vi "Engineering mode.vi"() -> ()   [LabVIEW 2017]
uses:
  Ctrls/TesterInfo.ctl
  Ctrls/HD Config.ctl
  Ctrls/AllControls.ctl
  Ctrls/Position Config.ctl
  <vilib>/Utility/miscctls.llb/LVRowAndColumnTypeDef.ctl
  DIPC 692 Daemon API/typdef/destination.ctl
  DIPC 692 Daemon API/typdef/device_mode.ctl
  ComVIS/Files/Ini/WriteIniFiles_ByVarient.vi
  <vilib>/Utility/file.llb/Write Delimited Spreadsheet (string).vi
  HardWare/ADLINK/IO/Adlink IO/Adlink IO.lvlib
panel:
  in  "Data":string
  out "Size":i32
  in  "AllControls":T1
  in  "Production Mode":bool
  out "Save_status":string
  in  "Selecttion":T2(tab)
  in  "HD Config Save":bool
  in  "HD Config":T3
  in  "SW Config Save":bool
  in  "TesterInfo":T4
  in  "Table":T5(tab)
  in  "Table_Data":string[][](table)
  in  "Title_Data":string[][](table)
  in  "Config":string[][](table)
  in  "SKU_Table":string[][](table)
  in  "Debug":T6(tab)
  in  "IO":i32(listbox)
  in  "Reset":bool
  in  "Set_MaxSpeed":u32
  in  "Set_Speed":bool
  in  "Set_MoveSpeed":u16 max=100
  in  "Stop":bool
  in  "Servo_Off":bool
  in  "Servo_On":bool
  in  "Position Config":T7
  in  "PositionSelect":T8(ring)
  in  "Home":bool
  in  "Position Config Save":bool
  in  "GoPosition":bool
  in  "Zero pressure":bool
  out "Status":string
  out "Units":string
  out "Pressure":string
  in  "FCO Model5_Read":bool
  out "FCO Data":string
  in  "Relay_ON/OFF":bool
  in  "DC_Power_ON/OFF":bool
  in  "DC_Set":bool
  in  "DC":bool
  out "DC Power Data":string
  in  "Voltage":dbl min=0.0 max=25.0
  in  "Current":dbl min=0.0 max=48.0
  out "Measurement":dbl[](array[numeric])
  in  "PW3336":bool
  out "PW3336 Data":string
  out "Atmospheric Pressure":dbl
  in  "Lefoo":bool
  out "Lefoo Data":string
  out "UID":string
  out "temperature":dbl
  out "humidity":dbl
  in  "Read_NFC":bool
  out "DataTag":string
  out "Data Return":string
  in  "Set EOL":bool
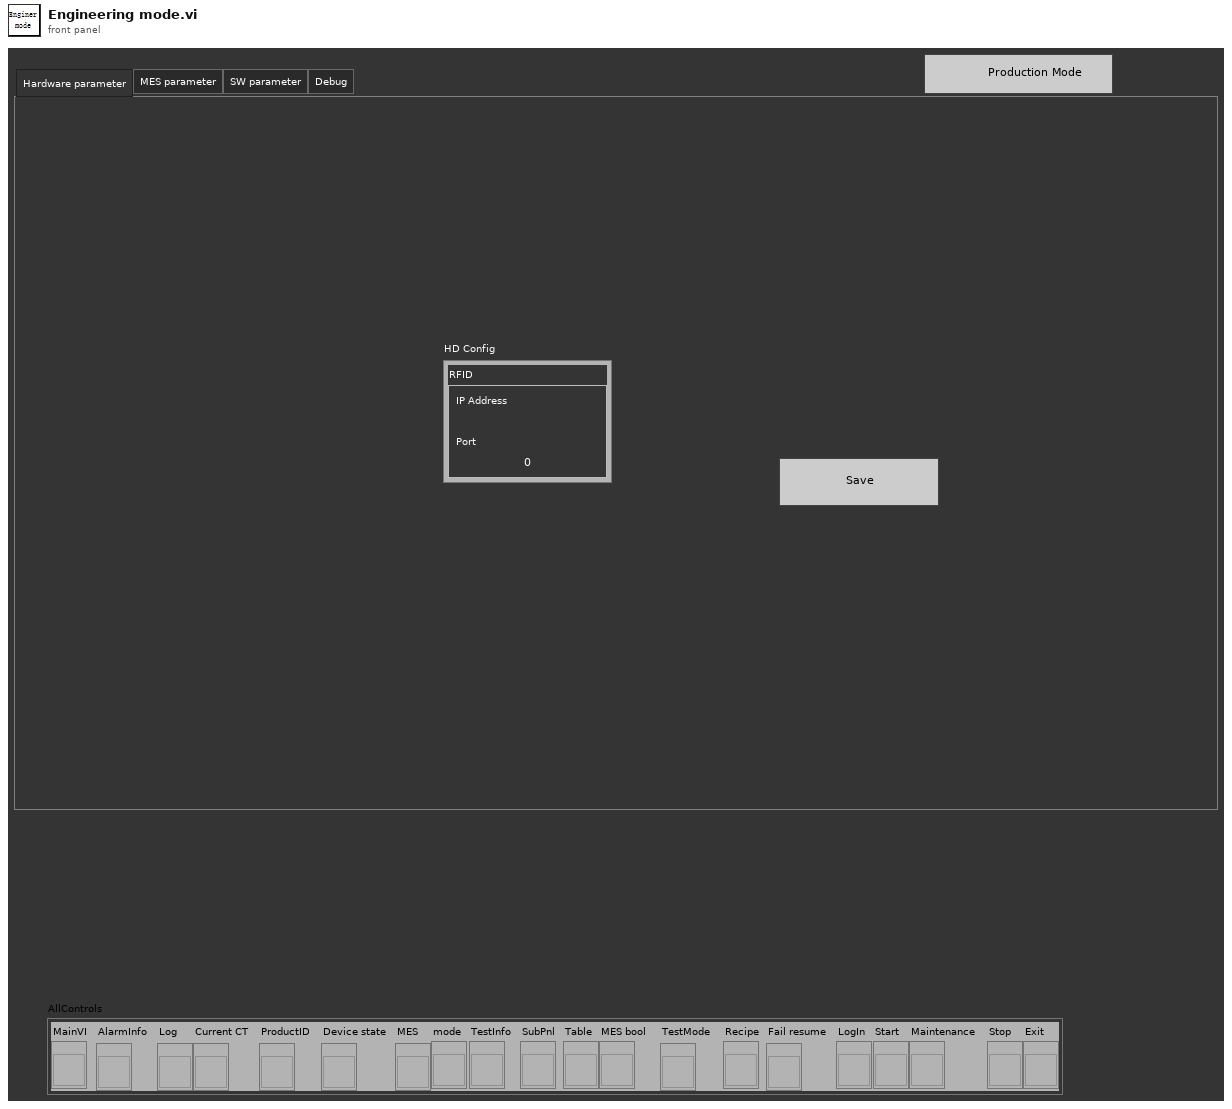
[diagram p1: front panel]
types:
  T1 = typedef "AllControls.ctl" = cluster{"MainVI":refnum<vi>, "AlarmInfo":refnum<vi>, "Log":refnum<vi>, "Current CT":refnum<vi>, "ProductID":refnum<vi>, "Device state":refnum<vi>, "MES":refnum<vi>, "mode":refnum<vi>, "TestInfo":refnum<vi>, "SubPnl":refnum<vi>, "Table":refnum<vi>, "MES bool":refnum<vi>, "TestMode":refnum<vi>, "Recipe":refnum<vi>, "Fail resume":refnum<vi>, "LogIn":refnum<vi>, "Start":refnum<vi>, "Maintenance":refnum<vi>, "Stop":refnum<vi>, "Exit":refnum<vi>}
  T2 = enum32{"Hardware parameter", "MES parameter", "SW parameter", "Debug"}
  T3 = typedef "HD Config.ctl" = cluster{" PC":cluster{"PC Address":u8[], "PC Port":i32}, "FCO":cluster{"COM":refnum<visa-resource-name>, "Baudrate":u32}, "DC Power ":cluster{"COM":refnum<visa-resource-name>, "Baudrate":u32}, "PW3336":cluster{"COM":refnum<visa-resource-name>, "Baudrate":u32}, "Lefoo":cluster{"COM":refnum<visa-resource-name>, "Baudrate":u32}, "AI Model":cluster{"COM":refnum<visa-resource-name>, "Baudrate":u32}, "DIPC":cluster{"COM":refnum<visa-resource-name>}, "RFID":cluster{"IP Address":string, "Port":u16, "Retry":u16}, "Motor":cluster{"COM":refnum<visa-resource-name>, "Baudrate":u32}, "Fail_resume_mode":bool, "GRR":bool}
  T4 = typedef "TesterInfo.ctl" = cluster{"Station Name":string, "Station Code":string, "ES NO.":string, "Tester ID":string, "PassMark Revision":string, "Rig ID":string, "Deamon_vision":string, "Project Name":string, "FFTesterPath":path, "Enable_User":bool, "Mode":enum16{"682"}, "MES":bool}
  T5 = enum32{"Process_parameter_Setting", "Title&Passmark_Setting", "Setting_Config", "SKU_Table"}
  T6 = enum32{"IO Control", "Motor_Plate control", "FCO_Pressure transmitter", "DC Power Supply ", "PW3336_Power Meter", "Lefoo_Atm Pressure", "RFID", "Set EOL_URAT"}
  T7 = typedef "Position Config.ctl" = cluster{"OrificeSize_12.7":i32, "OrificeSize_13":i32, "OrificeSize_30":i32, "OrificeSize_16":i32}
  T8 = enum16{"OrificeSize_12.7", "OrificeSize_13", "OrificeSize_30", "OrificeSize_16"}
  T9 = cluster{"DI dev":i32[], "DI line":i32[], "Port":i32[], "DO dev":i32[], "DO line":i32[], "IO Data":string[][], "IO f":i16[]}
  T10 = typedef "amc_Message Queue.ctl" = refnum<queue>
  T11 = enum8{"Enabled", "Disabled", "Disabled and Grayed Out"}
  T12 = typedef "LVRowAndColumnTypeDef.ctl" = cluster{"Row":i32, "Column":i32}
  T13 = typedef "device_mode.ctl" = enum16{"FCT", "EOL", "PROD"}
  T14 = typedef "destination.ctl" = string
  T15 = typedef "LVPoint32TypeDef.ctl" = cluster{"Horizontal":i32, "Vertical":i32}
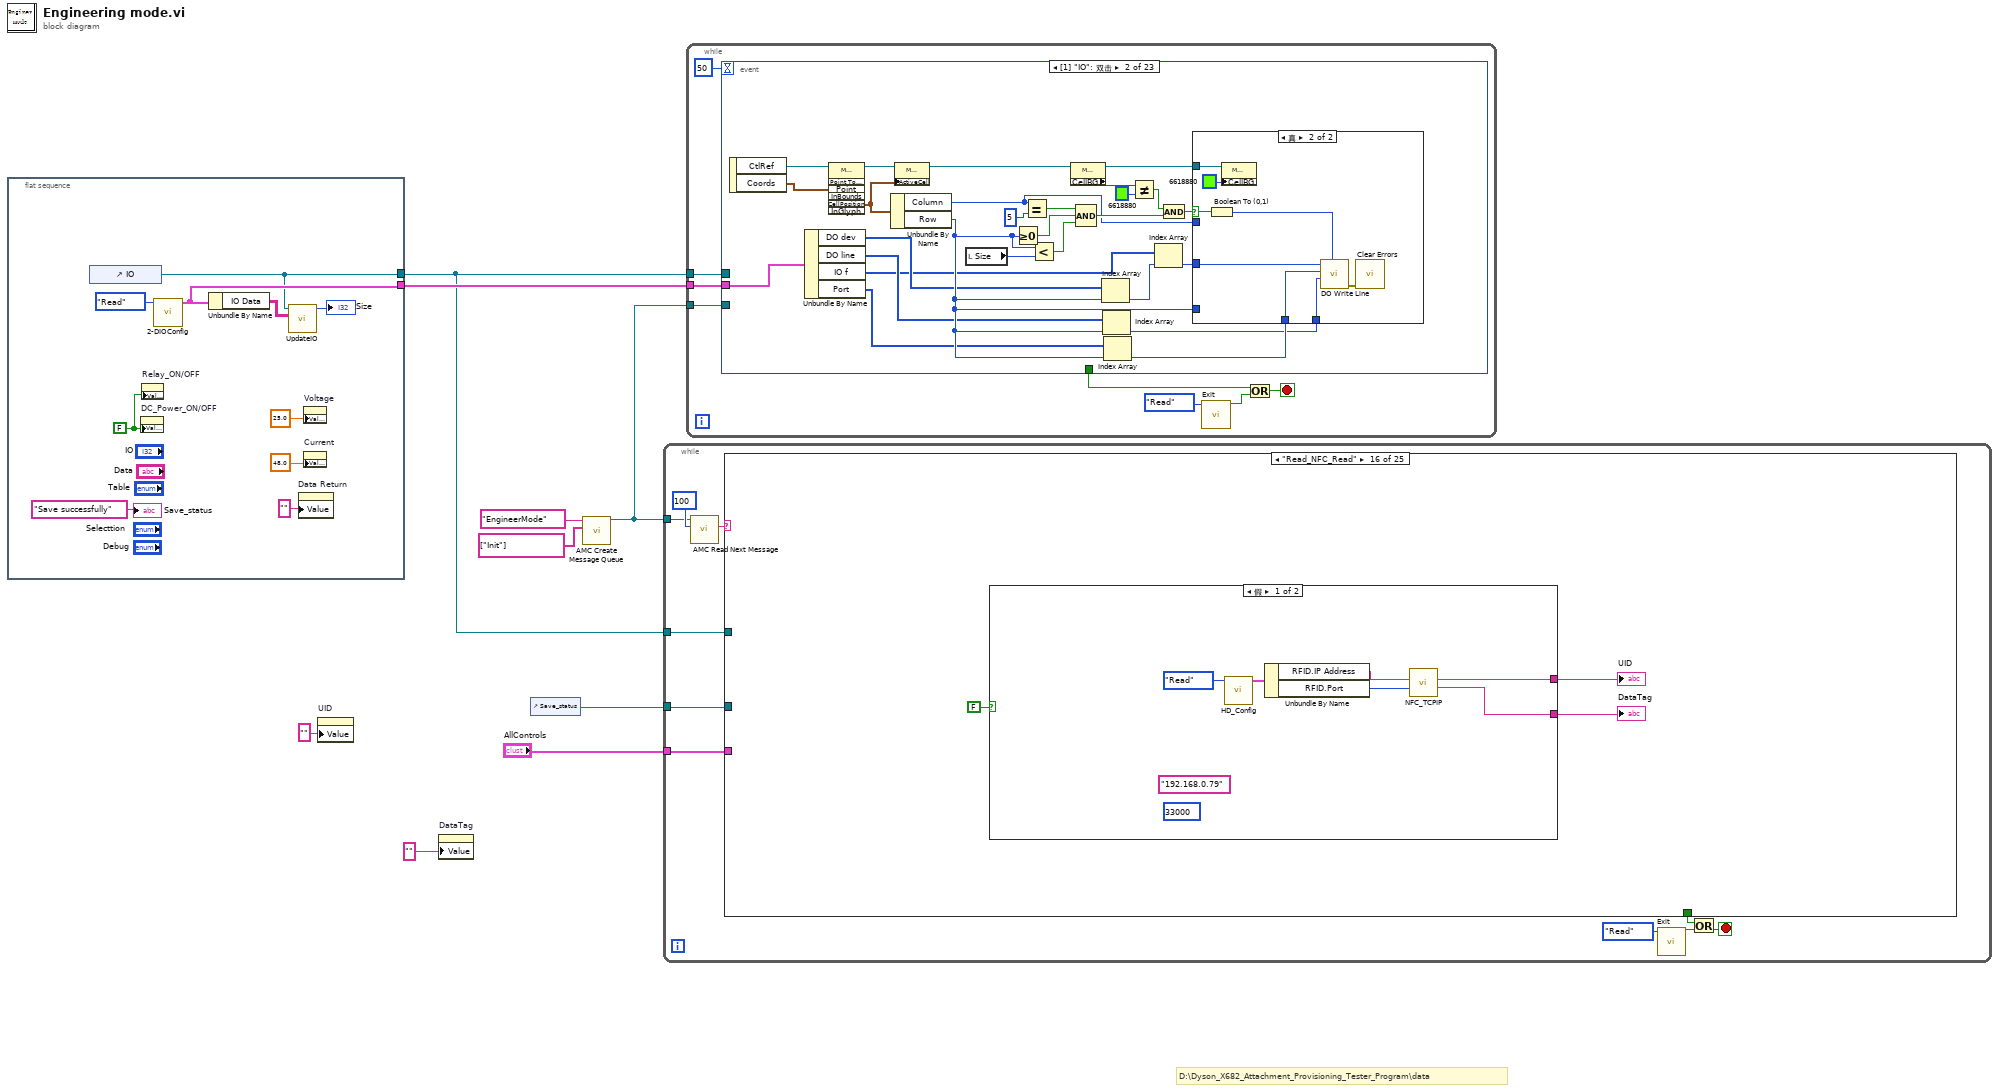
[diagram p0: block diagram]
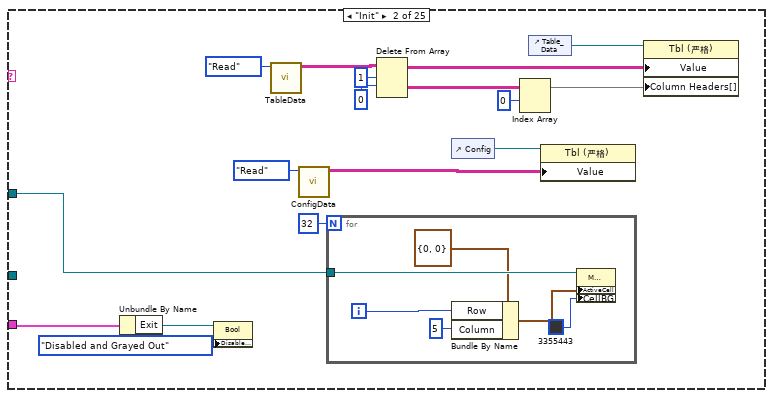
[diagram p3: hidden frame]
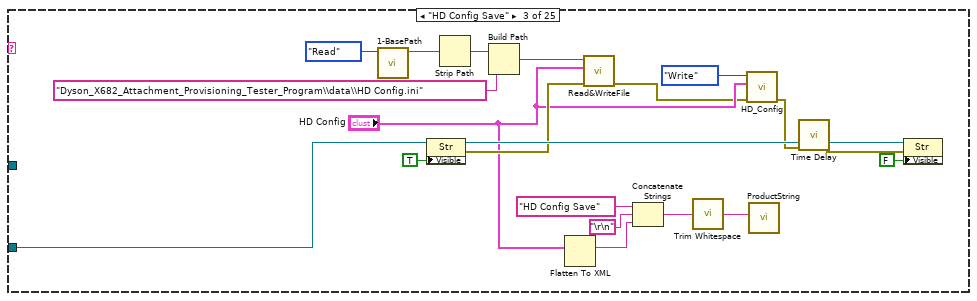
[diagram p4: hidden frame]
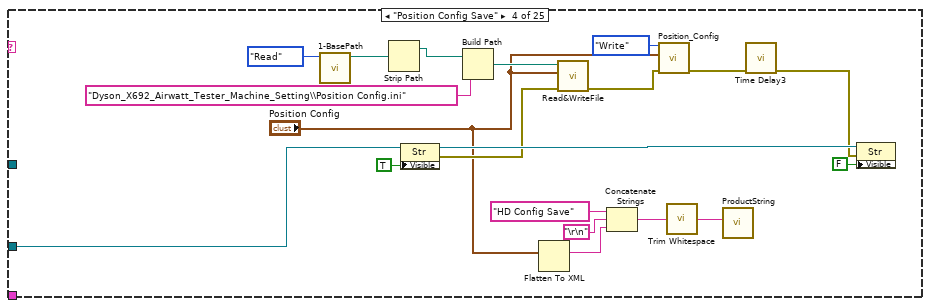
[diagram p5: hidden frame]
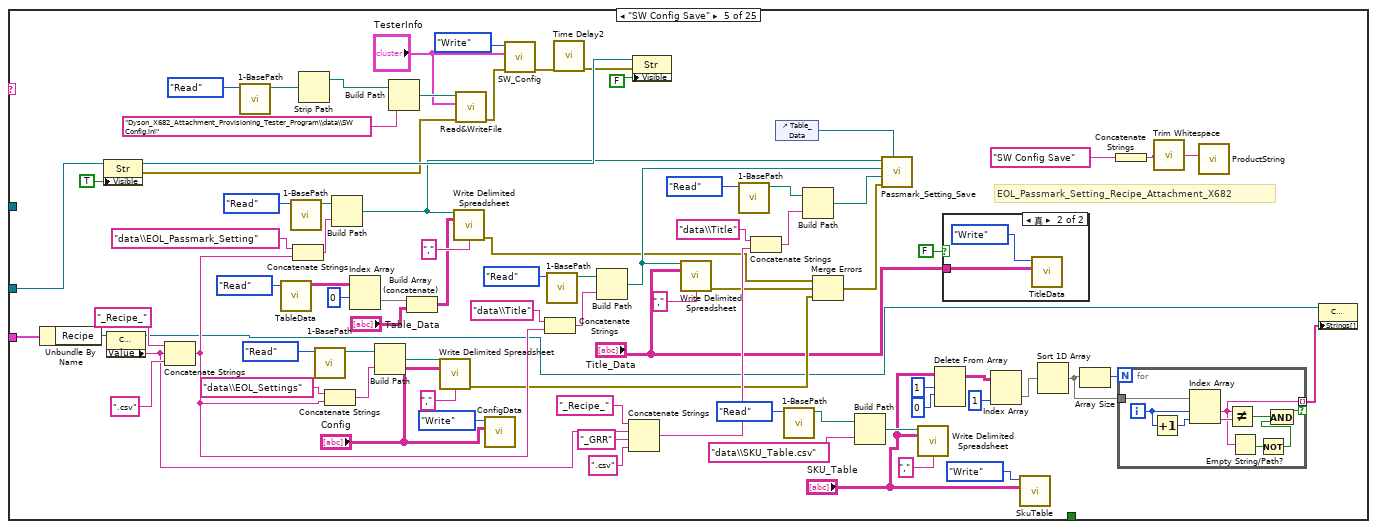
[diagram p6: hidden frame]
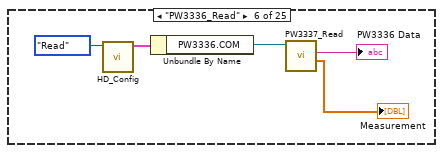
[diagram p8: hidden frame]
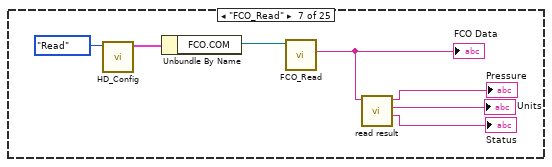
[diagram p9: hidden frame]
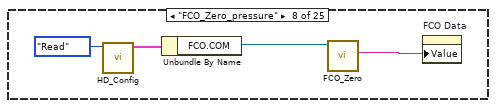
[diagram p10: hidden frame]
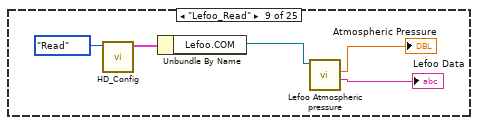
[diagram p11: hidden frame]
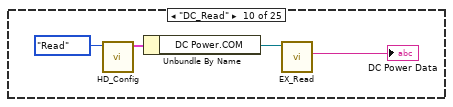
[diagram p12: hidden frame]
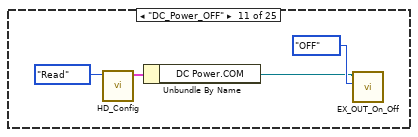
[diagram p13: hidden frame]
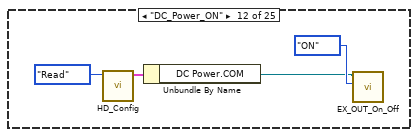
[diagram p14: hidden frame]
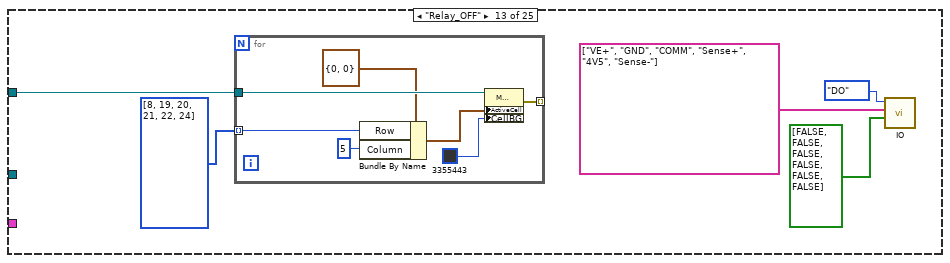
[diagram p15: hidden frame]
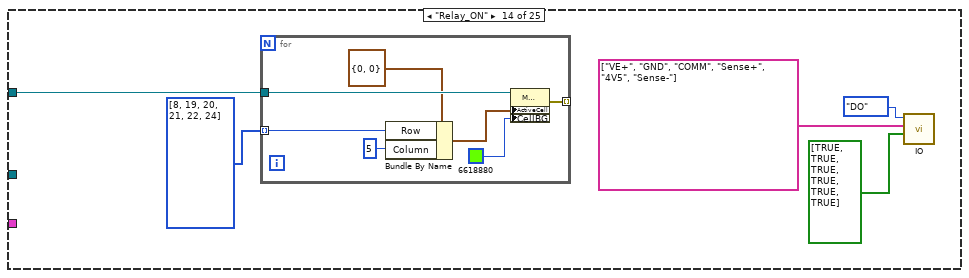
[diagram p16: hidden frame]
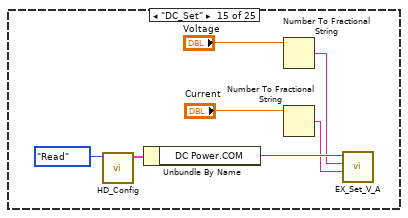
[diagram p17: hidden frame]
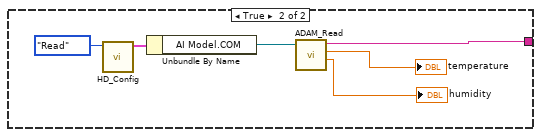
[diagram p18: hidden frame]
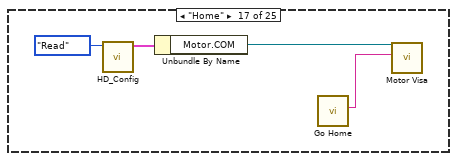
[diagram p19: hidden frame]
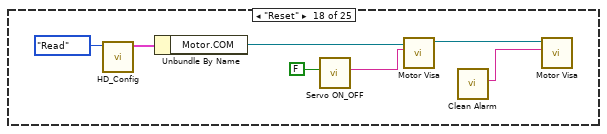
[diagram p20: hidden frame]
diagram:
  # "D:\\Dyson_X682_Attachment_Provisioning_Tester_Program\\data"
  n1 = flat-sequence {
    tunnel: [w17] -> w4
    tunnel: [w15] -> w3
    frame #0 {
      w10 = FALSE ("DC_Power_ON/OFF")
      n2 = control-ref of="IO"() -> (w15:refnum<vi>)
      n3 = property on="DC_Power_ON/OFF" class="Bool (strict)"("Value"=w10) -> ()  [unwired: 2 in, 2 out]
      n4 = property on="Relay_ON/OFF" class="Bool (严格)"("Value"=w10) -> ()  [unwired: 2 in, 2 out]
      n5 = call "2-DIOConfig.vi"("Step"=enum16{"Initial", "Write", "Read"}."Read") -> ("DIO pra out"=w17:T9)  [unwired: 9 in, 1 out]
      n6 = Unbundle By Name(w17) -> ("IO Data"=w16:string[][])
      n7 = call "UpdateIO.vi"("IO Data"=w16, "MulticolumnListbox输入"=w15) -> ("大小"=→"Size":i32)  [unwired: 9 in]
      n8 = property on="Data Return" class="Str"("Value"="" ("Data Return")) -> ()  [unwired: 2 in, 2 out]
      n9 = property on="Voltage" class="DigNum (strict)"("Value"=25.0 ("Voltage")) -> ()  [unwired: 2 in, 2 out]
      n10 = property on="Current" class="DigNum (strict)"("Value"=48.0 ("Current")) -> ()  [unwired: 2 in, 2 out]
      "Save_status" <- "Save successfully" ("Save_status")
    }
  }
  n11 = property on="UID" class="Str"("Value"="" ("UID")) -> ()  [unwired: 2 in, 2 out]
  n12 = property on="DataTag" class="Str"("Value"="") -> ()  [unwired: 2 in, 2 out]
  n13 = control-ref of="Save_status"() -> (w7:refnum<vi>)
  n14 = call "AMC Create Message Queue.vi"("Initial Message Names"=string[] ["Init"], "Message Queue Name"="EngineerMode" ("Message queue name (unnamed)")) -> ("Message Queue out"=w8:T10)  [unwired: 3 in, 6 out]
  n15 = while {
    tunnel: w8 -> [w26]
    tunnel: w7 -> [w22]
    tunnel: "AllControls" -> [w21]
    tunnel: w3 -> [w20]
    stop <- w24 stop-if-true
    n16 = call "AMC Read Next Message.vi"("timeout (1ms)"=100 ("Timeout"), "Message Queue in"=w26) -> ("Message Name"=w25:string)  [unwired: 2 in, 7 out]
    n17 = case shown="\"Read_NFC_Read\"" w25 {
      tunnel: [_ _ _ _ _ _ _ _ _ _ _ _ _ _ _ _ _ _ _ _ _ _ _ _ TRUE] -> w23
      tunnel: w22 -> [_ _ w63 w83 w171 _ _ _ _ _ _ _ _ _ _ _ _ _ _ _ _ _ _ _ _]
      tunnel: w21 -> [_ w32 _ _ w141 _ _ _ _ _ _ _ _ _ _ _ _ _ _ _ _ _ _ _ w371]
      tunnel: w20 -> [_ w33 _ _ _ _ _ _ _ _ _ _ w223 w234 _ _ _ _ _ _ _ _ _ _ w376]
      frame "假", Default {
      }
      frame "Init" {
        n18 = Unbundle By Name(w32) -> ("Exit"=w31:refnum<vi>)
        n19 = property class="Bool"(reference=w31, "DisabledEnum"=T11."Disabled and Grayed Out" ("Disabled")) -> ()  [unwired: 1 in, 2 out]
        n20 = call "TableData.vi"("Step"=enum16{"Initial", "Write", "Read"}."Read") -> ("Tabledata Out"=w42:string[][])  [unwired: 9 in, 1 out]
        n21 = call "ConfigData.vi"("Step"=enum16{"Initial", "Write", "Read"}."Read") -> ("Tabledata Out"=w35:string[][])  [unwired: 9 in, 1 out]
        n22 = for {
          N: 32 -> [_]
          tunnel: w33 -> [w52]
          i -> [w48]
          n23 = Bundle By Name(cluster=T12 {"Row"=0, "Column"=0} ("Active Cell:Active Cell"), "Row"=w48, "Column"=5) -> (w49:T12)
          n24 = property class="MCListbox (严格)"(reference=w52, "ActiveCell"=w49, "CellBG"=u32 3355443) -> ()  [unwired: 1 in, 2 out]
        }
        n25 = Delete From Array(array=w42, length=1 ("长度"), index (row)=0 ("索引 (行)")) -> (deleted portion=w40:string[][], array with subset deleted=w41:string[][])  [unwired: 1 in]
        n26 = control-ref of="Config"() -> (w36:refnum<vi>)
        n27 = Index Array(array=w40, index (row)=0 ("索引 (行)")) -> (element=w39:string[])  [unwired: 1 in]
        n28 = control-ref of="Table_Data"() -> (w46:refnum<vi>)
        n29 = property on="属性节点" class="Tbl (严格)"(reference=w36, "Value"=w35) -> ()  [unwired: 1 in, 2 out]
        n30 = property on="属性节点" class="Tbl (严格)"(reference=w46, "Value"=w41, "Column Headers[]"=w39) -> ()  [unwired: 1 in, 2 out]
      }
      frame "HD Config Save" {
        n31 = call "1-BasePath.vi"("Step"=enum16{"Initial", "Write", "Read"}."Read") -> ("Path Out"=w71:path)  [unwired: 9 in, 1 out]
        n32 = property class="Str"(reference=w63, "Visible"=TRUE ("可见")) -> (reference out=w66:refnum<vi>, error out=w65:errorcluster)  [unwired: 1 in]
        n33 = Strip Path(path=w71) -> (stripped path=w53:path)  [unwired: 1 out]
        n34 = Build Path(base path=w53, name or relative path="Dyson_X682_Attachment_Provisioning_Tester_Program\\data\\HD Config.ini") -> (appended path=w69:path)
        n35 = Flatten To XML(anything="HD Config") -> (xml string=w61:string)
        n36 = call-poly "Read&WriteFile.vi"("error in (no error)"=w65, "Variant"="HD Config", "path"=w69) -> ("error out"=w55:errorcluster)  [unwired: 8 in]
        n37 = Concatenate Strings("HD Config Save" ("String"), "\r\n", w61) -> (w62:string)
        n38 = call <vilib>:"Trim Whitespace.vi"("string"=w62) -> ("trimmed string"=w59:string)  [unwired: 1 in]
        n39 = call "HD_Config.vi"("error in (no error)"=w55, "HD Config in"="HD Config", "Step"=enum16{"Initial", "Write", "Read"}."Write") -> ("error out"=w54:errorcluster)  [unwired: 7 in, 1 out]
        n40 = call "ProductString.vi"("String"=w59) -> ()  [unwired: 10 in, 1 out]
        n41 = call "Time Delay"("error in (no error)"=w54) -> ("error out"=w56:errorcluster)  [unwired: 10 in]
        n42 = property class="Str"(reference=w66, error in=w56, "Visible"=FALSE ("可见")) -> ()  [unwired: 2 out]
      }
      frame "Position Config Save" {
        n43 = call "1-BasePath.vi"("Step"=enum16{"Initial", "Write", "Read"}."Read") -> ("Path Out"=w91:path)  [unwired: 9 in, 1 out]
        n44 = Strip Path(path=w91) -> (stripped path=w73:path)  [unwired: 1 out]
        n45 = property class="Str"(reference=w83, "Visible"=TRUE ("可见")) -> (reference out=w86:refnum<vi>, error out=w85:errorcluster)  [unwired: 1 in]
        n46 = Build Path(base path=w73, name or relative path="Dyson_X692_Airwatt_Tester_Machine_Setting\\Position Config.ini") -> (appended path=w89:path)
        n47 = Flatten To XML(anything="Position Config") -> (xml string=w81:string)
        n48 = call-poly "Read&WriteFile.vi"("error in (no error)"=w85, "Variant"="Position Config", "path"=w89) -> ("error out"=w76:errorcluster)  [unwired: 8 in]
        n49 = Concatenate Strings("HD Config Save" ("String"), "\r\n", w81) -> (w82:string)
        n50 = call "Position_Config.vi"("error in (no error)"=w76, "Position Config"="Position Config", "Step"=enum16{"Initial", "Write", "Read"}."Write") -> ("error out"=w75:errorcluster)  [unwired: 7 in, 1 out]
        n51 = call <vilib>:"Trim Whitespace.vi"("string"=w82) -> ("trimmed string"=w79:string)  [unwired: 1 in]
        n52 = call "ProductString.vi"("String"=w79) -> ()  [unwired: 10 in, 1 out]
        n53 = call "Time Delay3"("error in (no error)"=w75) -> ("error out"=w74:errorcluster)  [unwired: 10 in]
        n54 = property class="Str"(reference=w86, error in=w74, "Visible"=FALSE ("可见")) -> ()  [unwired: 2 out]
      }
      frame "SW Config Save" {
        # "EOL_Passmark_Setting_Recipe_Attachment_X682"
        n55 = Unbundle By Name(w141) -> ("Recipe"=w101:refnum<vi>)
        n56 = property class="Str"(reference=w171, "Visible"=TRUE ("可见")) -> (reference out=w173:refnum<vi>, error out=w163:errorcluster)  [unwired: 1 in]
        n57 = property class="CmbBox"(reference=w101) -> (reference out=w100:refnum<vi>, "Value"=w123:string)  [unwired: 1 in, 1 out]
        n58 = Concatenate Strings("_Recipe_" ("字符串"), w123, ".csv" ("字符串")) -> (w132:string)
        n59 = call "1-BasePath.vi"("Step"=enum16{"Initial", "Write", "Read"}."Read") -> ("Path Out"=w114:path)  [unwired: 9 in, 1 out]
        n60 = call "TableData.vi"("Step"=enum16{"Initial", "Write", "Read"}."Read") -> ("Tabledata Out"=w153:string[][])  [unwired: 9 in, 1 out]
        n61 = call "1-BasePath.vi"("Step"=enum16{"Initial", "Write", "Read"}."Read") -> ("Path Out"=w159:path)  [unwired: 9 in, 1 out]
        n62 = Concatenate Strings("data\\EOL_Passmark_Setting" ("name or relative path"), w132) -> (w137:string)
        n63 = Strip Path(path=w114) -> (stripped path=w113:path)  [unwired: 1 out]
        n64 = call "1-BasePath.vi"("Step"=enum16{"Initial", "Write", "Read"}."Read") -> ("Path Out"=w147:path)  [unwired: 9 in, 1 out]
        n65 = Concatenate Strings("data\\EOL_Settings" ("name or relative path"), w132) -> (w135:string)
        n66 = Build Path(base path=w159, name or relative path=w137) -> (appended path=w131:path)
        n67 = Index Array ("索引数组")(array=w153, index (row)=0 ("索引 (行)")) -> (element=w152:string[])  [unwired: 1 in]
        n68 = Build Path(base path=w147, name or relative path=w135) -> (appended path=w149:path)
        n69 = Build Path(base path=w113, name or relative path="Dyson_X682_Attachment_Provisioning_Tester_Program\\data\\SW Config.ini") -> (appended path=w165:path)
        n70 = Build Array (concatenate)(w152, "Table_Data") -> (w156:string[][])
        n71 = call-poly <vilib>:"Write Delimited Spreadsheet.vi"("file path (dialog if empty)"=w149, "2D data"="Config", "delimiter (\\t)"="," ("delimiter (\\t)")) -> ("error out"=w116:errorcluster)  [unwired: 11 in, 1 out]
        n72 = call-poly <vilib>:"Write Delimited Spreadsheet.vi"("file path (dialog if empty)"=w131, "2D data"=w156, "delimiter (\\t)"="," ("delimiter (\\t)")) -> ("error out"=w115:errorcluster)  [unwired: 11 in, 1 out]
        n73 = call-poly "Read&WriteFile.vi"("error in (no error)"=w163, "Variant"="TesterInfo", "path"=w165) -> ("error out"=w162:errorcluster)  [unwired: 8 in]
        n74 = call "ConfigData.vi"("Tabledata in"="Config", "Step"=enum16{"Initial", "Write", "Read"}."Write") -> ()  [unwired: 8 in, 2 out]
        n75 = call "SW_Config.vi"("error in (no error)"=w162, "SW Config In"="TesterInfo", "Step"=enum16{"Initial", "Write", "Read"}."Write") -> ("error out"=w161:errorcluster)  [unwired: 7 in, 1 out]
        n76 = Concatenate Strings("data\\Title" ("name or relative path"), w132) -> (w133:string)
        n77 = call "1-BasePath.vi"("Step"=enum16{"Initial", "Write", "Read"}."Read") -> ("Path Out"=w143:path)  [unwired: 9 in, 1 out]
        n78 = call "Time Delay2"("error in (no error)"=w161) -> ("error out"=w145:errorcluster)  [unwired: 10 in]
        n79 = Build Path(base path=w143, name or relative path=w133) -> (appended path=w130:path)
        n80 = Concatenate Strings("_Recipe_" ("字符串"), w123, "_GRR" ("字符串"), ".csv" ("字符串")) -> (w120:string)
        n81 = property class="Str"(reference=w173, error in=w145, "Visible"=FALSE ("可见")) -> ()  [unwired: 2 out]
        n82 = call-poly <vilib>:"Write Delimited Spreadsheet.vi"("file path (dialog if empty)"=w130, "2D data"="Title_Data", "delimiter (\\t)"="," ("delimiter (\\t)")) -> ("error out"=w119:errorcluster)  [unwired: 11 in, 1 out]
        n83 = call "1-BasePath.vi"("Step"=enum16{"Initial", "Write", "Read"}."Read") -> ("Path Out"=w127:path)  [unwired: 9 in, 1 out]
        n84 = Concatenate Strings("data\\Title" ("name or relative path"), w120) -> (w129:string)
        n85 = control-ref of="Table_Data"() -> (w118:refnum<vi>)
        n86 = call "1-BasePath.vi"("Step"=enum16{"Initial", "Write", "Read"}."Read") -> ("Path Out"=w107:path)  [unwired: 9 in, 1 out]
        n87 = Build Path(base path=w127, name or relative path=w129) -> (appended path=w125:path)
        n88 = Merge Errors(w115, w119, w116) -> (w117:errorcluster)
        n89 = Build Path(base path=w107, name or relative path="data\\SKU_Table.csv") -> (appended path=w112:path)
        n90 = call "Passmark_Setting_Save.vi"("Table_Data 2"=w118, "error in (no error)"=w117, "GRR_Title_Setting_path"=w125, "Title_Setting_path"=w130, "Flow_Setting_path"=w131) -> ()  [unwired: 6 in, 1 out]
        n91 = call-poly <vilib>:"Write Delimited Spreadsheet.vi"("file path (dialog if empty)"=w112, "2D data"="SKU_Table", "delimiter (\\t)"="," ("delimiter (\\t)")) -> ()  [unwired: 11 in, 2 out]
        n92 = Delete From Array(array="SKU_Table", length=1 ("长度"), index (row)=0 ("索引 (行)")) -> (array with subset deleted=w106:string[][])  [unwired: 1 in, 1 out]
        n93 = case shown="真" FALSE {
          tunnel: "Title_Data" -> [_ w175]
          frame False {
          }
          frame True {
            n94 = call "TitleData.vi"("Tabledata in"=w175, "Step"=enum16{"Initial", "Write", "Read"}."Write") -> ()  [unwired: 8 in, 2 out]
          }
        }
        n95 = Index Array(array=w106, index (col)=1 ("禁用的索引 (列)")) -> (element=w99:string[])  [unwired: 1 in]
        n96 = call "SkuTable.vi"("Tabledata in"="SKU_Table", "Step"=enum16{"Initial", "Write", "Read"}."Write") -> ()  [unwired: 8 in, 2 out]
        n97 = Sort 1D Array(array=w99) -> (sorted array=w97:string[])
        n98 = Array Size(array=w97) -> (size(s)=w98:i32)
        n99 = Concatenate Strings("SW Config Save" ("String")) -> (w170:string)
        n100 = for {
          N: w98 -> [_]
          tunnel: w97 -> [w185]
          tunnel: [w180] -> w96 mode=indexing if=w178
          i -> [w183]
          n101 = Increment(x=w183) -> (x+1=w182:i32)
          n102 = Index Array(array=w185, index #1=w183, index #2=w182) -> (element #1=w180:string, element #2=w181:string)
          n103 = Not Equal?(x=w180, y=w181) -> (x != y?=w184:bool)
          n104 = Empty String/Path?(string/path=w180) -> (empty?=w179:bool)
          n105 = Not(x=w179) -> (.not. x?=w177:bool)
          n106 = And(x=w184, y=w177) -> (x .and. y?=w178:bool)
        }
        n107 = call <vilib>:"Trim Whitespace.vi"("string"=w170) -> ("trimmed string"=w169:string)  [unwired: 1 in]
        n108 = call "ProductString.vi"("String"=w169) -> ()  [unwired: 10 in, 1 out]
        n109 = property class="CmbBox"(reference=w100, "Strings[]"=w96) -> ()  [unwired: 1 in, 2 out]
      }
      frame "PW3336_Read" {
        n110 = call "HD_Config.vi"("Step"=enum16{"Initial", "Write", "Read"}."Read") -> ("HD Config out"=w189:T3)  [unwired: 9 in, 1 out]
        n111 = Unbundle By Name(w189) -> ("PW3336.COM"=w187:refnum<visa-resource-name>)
        n112 = call "PW3337_Read.vi"("VISA resource name"=w187) -> ("Measurement out"=→"Measurement":dbl[], "读取缓冲区"=→"PW3336 Data":string)  [unwired: 7 in, 2 out]
      }
      frame "FCO_Read" {
        n113 = call "HD_Config.vi"("Step"=enum16{"Initial", "Write", "Read"}."Read") -> ("HD Config out"=w197:T3)  [unwired: 9 in, 1 out]
        n114 = Unbundle By Name(w197) -> ("FCO.COM"=w195:refnum<visa-resource-name>)
        n115 = call "FCO_Read.vi"("VISA in"=w195) -> ("data"=w194:string)  [unwired: 7 in, 3 out]
        "FCO Data" <- w194
        n116 = call "read result.vi"("string in"=w194) -> ("Status"=→"Status":string, "Units"=→"Units":string, "Pressure"=→"Pressure":string)  [unwired: 8 in]
      }
      frame "FCO_Zero_pressure" {
        n117 = call "HD_Config.vi"("Step"=enum16{"Initial", "Write", "Read"}."Read") -> ("HD Config out"=w201:T3)  [unwired: 9 in, 1 out]
        n118 = Unbundle By Name(w201) -> ("FCO.COM"=w199:refnum<visa-resource-name>)
        n119 = call "FCO_Zero.vi"("VISA in"=w199) -> ("data"=w198:string)  [unwired: 8 in, 2 out]
        n120 = property on="FCO Data" class="Str"("Value"=w198) -> ()  [unwired: 2 in, 2 out]
      }
      frame "Lefoo_Read" {
        n121 = call "HD_Config.vi"("Step"=enum16{"Initial", "Write", "Read"}."Read") -> ("HD Config out"=w206:T3)  [unwired: 9 in, 1 out]
        n122 = Unbundle By Name(w206) -> ("Lefoo.COM"=w204:refnum<visa-resource-name>)
        n123 = call "Lefoo Atmospheric pressure.vi"("VISA resource name"=w204) -> ("data"=→"Lefoo Data":string, "Atmospheric pressure"=→"Atmospheric Pressure":dbl)  [unwired: 8 in, 1 out]
      }
      frame "DC_Read" {
        n124 = call "HD_Config.vi"("Step"=enum16{"Initial", "Write", "Read"}."Read") -> ("HD Config out"=w210:T3)  [unwired: 9 in, 1 out]
        n125 = Unbundle By Name(w210) -> ("DC Power.COM"=w207:refnum<visa-resource-name>)
        n126 = call "EX_Read.vi"("VISA resource name"=w207) -> ("读取缓冲区"=→"DC Power Data":string)  [unwired: 8 in, 2 out]
      }
      frame "DC_Power_OFF" {
        n127 = call "HD_Config.vi"("Step"=enum16{"Initial", "Write", "Read"}."Read") -> ("HD Config out"=w214:T3)  [unwired: 9 in, 1 out]
        n128 = Unbundle By Name(w214) -> ("DC Power.COM"=w211:refnum<visa-resource-name>)
        n129 = call "EX_OUT_On_Off.vi"("Mode"=enum16{"ON", "OFF"}."OFF", "VISA resource name"=w211) -> ()  [unwired: 8 in, 2 out]
      }
      frame "DC_Power_ON" {
        n130 = call "HD_Config.vi"("Step"=enum16{"Initial", "Write", "Read"}."Read") -> ("HD Config out"=w218:T3)  [unwired: 9 in, 1 out]
        n131 = Unbundle By Name(w218) -> ("DC Power.COM"=w215:refnum<visa-resource-name>)
        n132 = call "EX_OUT_On_Off.vi"("Mode"=enum16{"ON", "OFF"}."ON", "VISA resource name"=w215) -> ()  [unwired: 8 in, 2 out]
      }
      frame "Relay_OFF" {
        n133 = for {
          tunnel: w223 -> [w230]
          tunnel: [w225] -> _ mode=indexing
          tunnel: i32[] [8, 19, 20, 21, 22, 24] -> [w224] mode=indexing
          n134 = Bundle By Name(cluster=T12 {"Row"=0, "Column"=0} ("Active Cell:Active Cell"), "Row"=w224, "Column"=5) -> (w227:T12)
          n135 = property class="MCListbox (严格)"(reference=w230, "ActiveCell"=w227, "CellBG"=u32 3355443) -> (error out=w225:errorcluster)  [unwired: 1 in, 1 out]
        }
        n136 = call "IO.vi"("DO DATA"=bool[] [FALSE, FALSE, FALSE, FALSE, FALSE, FALSE] ("Writel_IO"), "IO Name"=string[] ["VE+", "GND", "COMM", "Sense+", "4V5", "Sense-"], "IO?"=enum16{"DI", "DO"}."DO") -> ()  [unwired: 6 in, 3 out]
      }
      frame "Relay_ON" {
        n137 = for {
          tunnel: w234 -> [w242]
          tunnel: [w237] -> _ mode=indexing
          tunnel: i32[] [8, 19, 20, 21, 22, 24] -> [w236] mode=indexing
          n138 = Bundle By Name(cluster=T12 {"Row"=0, "Column"=0} ("Active Cell:Active Cell"), "Row"=w236, "Column"=5) -> (w239:T12)
          n139 = property class="MCListbox (严格)"(reference=w242, "ActiveCell"=w239, "CellBG"=u32 6618880) -> (error out=w237:errorcluster)  [unwired: 1 in, 1 out]
        }
        n140 = call "IO.vi"("DO DATA"=bool[] [TRUE, TRUE, TRUE, TRUE, TRUE, TRUE] ("Writel_IO"), "IO Name"=string[] ["VE+", "GND", "COMM", "Sense+", "4V5", "Sense-"], "IO?"=enum16{"DI", "DO"}."DO") -> ()  [unwired: 6 in, 3 out]
      }
      frame "DC_Set" {
        n141 = call "HD_Config.vi"("Step"=enum16{"Initial", "Write", "Read"}."Read") -> ("HD Config out"=w249:T3)  [unwired: 9 in, 1 out]
        n142 = Unbundle By Name(w249) -> ("DC Power.COM"=w247:refnum<visa-resource-name>)
        n143 = Number To Fractional String(number="Voltage") -> (F-format string=w246:string)  [unwired: 3 in]
        n144 = Number To Fractional String(number="Current") -> (F-format string=w245:string)  [unwired: 3 in]
        n145 = call "EX_Set_V_A.vi"("current"=w245, "voltage"=w246, "VISA resource name"=w247) -> ()  [unwired: 7 in, 2 out]
      }
      frame "Read_NFC_Read" {
        n146 = case shown="假" FALSE {
          tunnel: [w258 w261] -> w252
          tunnel: [w257 _] -> w250
          frame False {
            (unwired) u16 33000 ("port")
            (unwired) "192.168.0.79" ("IP")
            n147 = call "HD_Config.vi"("Step"=enum16{"Initial", "Write", "Read"}."Read") -> ("HD Config out"=w255:T3)  [unwired: 9 in, 1 out]
            n148 = Unbundle By Name(w255) -> ("RFID.IP Address"=w253:string, "RFID.Port"=w254:u16)
            n149 = call "NFC_TCPIP.vi"("port"=w254, "IP"=w253) -> ("Read Data"=w258:string, "UID"=w257:string)  [unwired: 8 in]
          }
          frame True {
            n150 = call "HD_Config.vi"("Step"=enum16{"Initial", "Write", "Read"}."Read") -> ("HD Config out"=w264:T3)  [unwired: 9 in, 1 out]
            n151 = Unbundle By Name(w264) -> ("AI Model.COM"=w262:refnum<visa-resource-name>)
            n152 = call "ADAM_Read.vi"("VISA resource name"=w262) -> ("humidity"=→"humidity":dbl, "temperature"=→"temperature":dbl, "Data"=w261:string)  [unwired: 7 in, 1 out]
          }
        }
        "DataTag" <- w252
        "UID" <- w250
      }
      frame "Home" {
        n153 = call "HD_Config.vi"("Step"=enum16{"Initial", "Write", "Read"}."Read") -> ("HD Config out"=w268:T3)  [unwired: 9 in, 1 out]
        n154 = Unbundle By Name(w268) -> ("Motor.COM"=w265:refnum<visa-resource-name>)
        n155 = call "Go Home.vi"() -> ("Go Home"=w266:string)  [unwired: 11 in]
        n156 = call "Motor Visa.vi"("Command"=w266, "VISA资源名称"=w265) -> ()  [unwired: 7 in, 3 out]
      }
      frame "Reset" {
        n157 = call "HD_Config.vi"("Step"=enum16{"Initial", "Write", "Read"}."Read") -> ("HD Config out"=w275:T3)  [unwired: 9 in, 1 out]
        n158 = Unbundle By Name(w275) -> ("Motor.COM"=w270:refnum<visa-resource-name>)
        n159 = call "Servo ON_OFF.vi"("Servo ON/OFF"=FALSE) -> ("Command"=w271:string)  [unwired: 10 in]
        n160 = call "Motor Visa.vi"("Command"=w271, "VISA资源名称"=w270) -> ("VISA资源名称输出"=w269:refnum<visa-resource-name>)  [unwired: 7 in, 2 out]
        n161 = call "Clean Alarm.vi"() -> ("Clean Alarm"=w273:string)  [unwired: 11 in]
        n162 = call "Motor Visa.vi"("Command"=w273, "VISA资源名称"=w269) -> ()  [unwired: 7 in, 3 out]
      }
      frame "Stop" {
        n163 = call "HD_Config.vi"("Step"=enum16{"Initial", "Write", "Read"}."Read") -> ("HD Config out"=w279:T3)  [unwired: 9 in, 1 out]
        n164 = Unbundle By Name(w279) -> ("Motor.COM"=w276:refnum<visa-resource-name>)
        n165 = call "Stop Command.vi"() -> ("Stop"=w277:string)  [unwired: 11 in]
        n166 = call "Motor Visa.vi"("Command"=w277, "VISA资源名称"=w276) -> ()  [unwired: 7 in, 3 out]
      }
      frame "Servo_On" {
        n167 = call "HD_Config.vi"("Step"=enum16{"Initial", "Write", "Read"}."Read") -> ("HD Config out"=w284:T3)  [unwired: 9 in, 1 out]
        n168 = Unbundle By Name(w284) -> ("Motor.COM"=w281:refnum<visa-resource-name>)
        n169 = call "Servo ON_OFF.vi"("Servo ON/OFF"=TRUE) -> ("Command"=w282:string)  [unwired: 10 in]
        n170 = call "Motor Visa.vi"("Command"=w282, "VISA资源名称"=w281) -> ()  [unwired: 7 in, 3 out]
      }
      frame "Servo_Off" {
        n171 = call "HD_Config.vi"("Step"=enum16{"Initial", "Write", "Read"}."Read") -> ("HD Config out"=w289:T3)  [unwired: 9 in, 1 out]
        n172 = Unbundle By Name(w289) -> ("Motor.COM"=w286:refnum<visa-resource-name>)
        n173 = call "Servo ON_OFF.vi"("Servo ON/OFF"=FALSE) -> ("Command"=w285:string)  [unwired: 10 in]
        n174 = call "Motor Visa.vi"("Command"=w285, "VISA资源名称"=w286) -> ()  [unwired: 7 in, 3 out]
      }
      frame "Set_Speed" {
        n175 = call "HD_Config.vi"("Step"=enum16{"Initial", "Write", "Read"}."Read") -> ("HD Config out"=w300:T3)  [unwired: 9 in, 1 out]
        n176 = To Long Integer(number="Set_MoveSpeed") -> (32bit integer=w291:i32)
        n177 = Unbundle By Name(w300) -> ("Motor.COM"=w298:refnum<visa-resource-name>)
        n178 = To Long Integer(number="Set_MaxSpeed") -> (32bit integer=w290:i32)
        n179 = call "Speed 0800.vi"("Speed"=w290) -> ("Command"=w293:string)  [unwired: 10 in]
        n180 = call "Speed.vi"("Speed"=w291) -> ("速度"=w292:string)  [unwired: 10 in]
        n181 = call "Motor Visa.vi"("Command"=w293, "VISA资源名称"=w298) -> ("错误输出"=w294:errorcluster, "VISA资源名称输出"=w295:refnum<visa-resource-name>)  [unwired: 7 in, 1 out]
        n182 = call "Motor Visa.vi"("错误输入（无错误）"=w294, "Command"=w292, "VISA资源名称"=w295) -> ()  [unwired: 6 in, 3 out]
      }
      frame "GoPosition" {
        n183 = property on="Position Config" class="Clust (严格)"() -> ("Value"=w307:T7)  [unwired: 2 in, 2 out]
        n184 = call "HD_Config.vi"("Step"=enum16{"Initial", "Write", "Read"}."Read") -> ("HD Config out"=w311:T3)  [unwired: 9 in, 1 out]
        n185 = case shown="\"OrificeSize_13\"" "PositionSelect" {
          tunnel: w307 -> [w313 w315 w317 w319]
          tunnel: [w312 w314 w316 w318] -> w306
          frame "OrificeSize_12.7", Default {
            n186 = Unbundle By Name(w313) -> ("OrificeSize_12.7"=w312:i32)
          }
          frame "OrificeSize_13" {
            n187 = Unbundle By Name(w315) -> ("OrificeSize_13"=w314:i32)
          }
          frame "OrificeSize_30" {
            n188 = Unbundle By Name(w317) -> ("OrificeSize_30"=w316:i32)
          }
          frame "OrificeSize_16" {
            n189 = Unbundle By Name(w319) -> ("OrificeSize_16"=w318:i32)
          }
        }
        n190 = Unbundle By Name(w311) -> ("Motor.COM"=w309:refnum<visa-resource-name>)
        n191 = To Long Integer(number=w306) -> (32bit integer=w302:i32)
        n192 = call "Pulse.vi"("Pulse"=w302) -> ("Pulse"=w303:string)  [unwired: 10 in]
        n193 = call "Motor Visa.vi"("Command"=w303, "VISA资源名称"=w309) -> ("错误输出"=w304:errorcluster, "VISA资源名称输出"=w305:refnum<visa-resource-name>)  [unwired: 7 in, 1 out]
        n194 = call "ABS.vi"() -> ("绝对模式"=w301:string)  [unwired: 11 in]
        n195 = call "Motor Visa.vi"("错误输入（无错误）"=w304, "Command"=w301, "VISA资源名称"=w305) -> ()  [unwired: 6 in, 3 out]
      }
      frame "Set_EOL" {
        n196 = call "HD_Config.vi"("Step"=enum16{"Initial", "Write", "Read"}."Read") -> ("HD Config out"=w362:T3)  [unwired: 9 in, 1 out]
        n197 = Unbundle By Name(w362) -> ("RFID.IP Address"=w360:string, "RFID.Port"=w359:u16, "DC Power.COM"=w325:refnum<visa-resource-name>, "DIPC.COM"=w351:refnum<visa-resource-name>)
        n198 = call "IO.vi"("DO DATA"=bool[] [TRUE] ("Writel_IO"), "IO Name"=string[] ["Probe_Cylinder"], "IO?"=enum16{"DI", "DO"}."DO") -> ("error out"=w367:errorcluster)  [unwired: 6 in, 2 out]
        n199 = call "Time Delay4"("error in (no error)"=w367) -> ("error out"=w363:errorcluster)  [unwired: 10 in]
        n200 = call "daemon connect.vi"("port (6543)"=w359, "address (localhost)"=w360) -> ("daemon reference out"=w347:refnum<k5>)  [unwired: 8 in, 1 out]
        n201 = call "IO.vi"("错误常量"=w363, "DO DATA"=bool[] [TRUE, TRUE, TRUE, TRUE, TRUE] ("Writel_IO"), "IO Name"=string[] ["VE+", "GND", "COMM", "WAKE", "4V5"], "IO?"=enum16{"DI", "DO"}."DO") -> ("error out"=w353:errorcluster)  [unwired: 5 in, 2 out]
        n202 = call "EX_Set_V_A.vi"("错误输入（无错误）"=w353, "current"="48", "voltage"="25", "VISA resource name"=w325) -> ("VISA资源名称输出"=w356:refnum<visa-resource-name>)  [unwired: 6 in, 1 out]
        n203 = call "EX_OUT_On_Off.vi"("Mode"=enum16{"ON", "OFF"}."ON", "VISA resource name"=w356) -> ("error out"=w354:errorcluster)  [unwired: 8 in, 1 out]
        n204 = call "Time Delay5"("error in (no error)"=w354) -> ("error out"=w350:errorcluster)  [unwired: 10 in]
        n205 = call "connect.vi"("error in (no error)"=w350, "Target"=T14 "DDM", "physical connection"=w351, "daemon reference in"=w347) -> ("error out"=w348:errorcluster, "response"=w338:string, "daemon reference out"=w346:refnum<k5>)  [unwired: 3 in, 2 out]
        n206 = call "Time Delay6"("error in (no error)"=w348) -> ("error out"=w340:errorcluster)  [unwired: 10 in]
        n207 = call "set_device_mode.vi"("error in (no error)"=w340, "Mode"=device_mode."EOL", "daemon reference in"=w346) -> ("error out"=w344:errorcluster, "response"=w339:string, "daemon reference out"=w345:refnum<k5>)  [unwired: 5 in, 1 out]
        n208 = Concatenate Strings(w338, "\n", w339) -> (→"Data Return":string)
        n209 = call "Time Delay7"("error in (no error)"=w344) -> ("error out"=w343:errorcluster)  [unwired: 10 in]
        n210 = call "disconnect.vi"("error in (no error)"=w343, "daemon reference in"=w345) -> ("error out"=w341:errorcluster, "daemon reference out"=w342:refnum<k5>)  [unwired: 6 in, 2 out]
        n211 = call "daemon disconnect.vi"("error in (no error)"=w341, "daemon reference in"=w342) -> ("error out"=w326:errorcluster)  [unwired: 9 in]
        n212 = call "EX_Set_V_A.vi"("错误输入（无错误）"=w326, "current"="0", "voltage"="0", "VISA resource name"=w325) -> ("error out"=w321:errorcluster, "VISA资源名称输出"=w334:refnum<visa-resource-name>)  [unwired: 6 in]
        n213 = call "EX_OUT_On_Off.vi"("错误输入（无错误）"=w321, "Mode"=enum16{"ON", "OFF"}."OFF", "VISA resource name"=w334) -> ("error out"=w333:errorcluster)  [unwired: 7 in, 1 out]
        n214 = call "Time Delay8"("error in (no error)"=w333) -> ("error out"=w335:errorcluster)  [unwired: 10 in]
        n215 = call "IO.vi"("错误常量"=w335, "DO DATA"=bool[] [FALSE, FALSE, FALSE, FALSE, FALSE] ("Writel_IO"), "IO Name"=string[] ["VE+", "GND", "COMM", "WAKE", "4V5"], "IO?"=enum16{"DI", "DO"}."DO") -> ("error out"=w320:errorcluster)  [unwired: 5 in, 2 out]
        n216 = call "IO.vi"("错误常量"=w320, "DO DATA"=bool[] [FALSE] ("Writel_IO"), "IO Name"=string[] ["Probe_Cylinder"], "IO?"=enum16{"DI", "DO"}."DO") -> ()  [unwired: 5 in, 3 out]
      }
      frame "PrductionMode" {
        n217 = for {
          N: 32 -> [_]
          tunnel: w376 -> [w384]
          tunnel: [w378] -> _ mode=indexing
          i -> [w380]
          n218 = Bundle By Name(cluster=T12 {"Row"=0, "Column"=0} ("Active Cell:Active Cell"), "Row"=w380, "Column"=5) -> (w381:T12)
          n219 = property class="MCListbox (严格)"(reference=w384, "ActiveCell"=w381, "CellBG"=u32 3355443) -> (error out=w378:errorcluster)  [unwired: 1 in, 1 out]
        }
        n220 = Unbundle By Name(w371) -> ("Exit"=w373:refnum<vi>)
        n221 = property class="Bool"(reference=w373, "DisabledEnum"=T11."Enabled" ("Disabled")) -> ()  [unwired: 1 in, 2 out]
        n222 = call "ProductString.vi"("String"="Return to production mode") -> ()  [unwired: 10 in, 1 out]
      }
    }
    n223 = call "Exit.vi"("Step"=enum16{"Initial", "Write", "Read"}."Read") -> ("Exit Out"=w29:bool)  [unwired: 9 in, 1 out]
    n224 = Or(x=w23, y=w29) -> (x .or. y?=w24:bool)
  }
  n225 = while {
    tunnel: w8 -> [w388]
    tunnel: w3 -> [w386]
    tunnel: w4 -> [w385]
    stop <- w391 stop-if-true
    n226 = event shown="[1] \"IO\": 双击" {
      selector: _ -> [_ _ _ _ _ _ _ _ _ _ _ _ _ _ _ _ _ _ _ _ _ _ _]
      dyn-events: _ -> [_ _ _ _ _ _ _ _ _ _ _ _ _ _ _ _ _ _ _ _ _ _ _]
      timeout: 50 -> [_ _ _ _ _ _ _ _ _ _ _ _ _ _ _ _ _ _ _ _ _ _ _]
      tunnel: w388 -> [_ _ w479 w488 w499 w509 w513 w523 w527 w533 w537 w541 w545 w556 w566 w576 w586 w596 w606 w616 w626 w636 w647]
      tunnel: [_ _ _ _ _ _ _ _ _ _ _ _ _ _ _ _ _ _ _ _ _ _ w646] -> w387
      tunnel: w386 -> [w393 _ _ _ _ _ _ _ _ _ _ _ _ _ _ _ _ _ _ _ _ _ _]
      tunnel: w385 -> [w394 w425 _ _ _ _ _ _ _ _ _ _ _ _ _ _ _ _ _ _ _ _ _]
      event Timeout {
        n227 = event-data() -> ()  [unwired: 1 in, 1 out]
        n228 = Unbundle By Name(w394) -> ("DI dev"=w395:i32[], "Port"=w396:i32[], "DI line"=w397:i32[], "IO f"=w398:i16[])
        n229 = for {
          tunnel: w393 -> [w399]
          tunnel: w395 -> [w402] mode=indexing
          tunnel: w397 -> [w405] mode=indexing
          tunnel: w396 -> [w403] mode=indexing
          tunnel: w398 -> [w400]
          i -> [w404]
          n230 = Index Array(array=w400, index=w402) -> (element=w401:i16)
          n231 = call "DI Read Line.vi"("Line"=w405, "Port"=w403, "CardNumber"=w401) -> ("error out"=w408:errorcluster, "State out"=w407:u16)  [unwired: 6 in, 1 out]
          n232 = Not Equal To 0?(x=w407) -> (x != 0?=w406:bool)
          n233 = call <vilib>:"Clear Errors.vi"("error in (no error)"=w408) -> ()  [unwired: 5 in, 2 out]
          n234 = case shown="真" w406 {
            tunnel: w404 -> [w410 w419]
            tunnel: w399 -> [w409 w416]
            frame False {
              n235 = Bundle By Name(cluster=T12 {"Row"=0, "Column"=0} ("活动单元格:活动单元格"), "Row"=w410, "Column"=2) -> (w413:T12)
              n236 = property class="MCListbox (严格)"(reference=w409, "ActiveCell"=w413) -> (reference out=w415:refnum<vi>)  [unwired: 1 in, 1 out]
              n237 = property class="MCListbox (严格)"(reference=w415, "CellBG"=u32 3355443) -> ()  [unwired: 1 in, 2 out]
            }
            frame True {
              n238 = Bundle By Name(cluster=T12 {"Row"=0, "Column"=0} ("活动单元格:活动单元格"), "Row"=w419, "Column"=2) -> (w420:T12)
              n239 = property class="MCListbox (严格)"(reference=w416, "ActiveCell"=w420) -> (reference out=w422:refnum<vi>)  [unwired: 1 in, 1 out]
              n240 = property class="MCListbox (严格)"(reference=w422, "CellBG"=u32 6618880) -> ()  [unwired: 1 in, 2 out]
            }
          }
        }
      }
      event "IO": Double Click {
        n241 = event-data() -> ("CtlRef"=w424:refnum<vi>, "Coords"=w423:T15)  [unwired: 1 in]
        n242 = Unbundle By Name(w425) -> ("DO dev"=w430:i32[], "DO line"=w429:i32[], "IO f"=w428:i16[], "Port"=w447:i32[])
        n243 = invoke class="MCListbox (严格)" method="Point To Row Column"(reference=w424, "Point"=w423) -> (reference out=w443:refnum<vi>, "CellPosition"=w434:T12)  [unwired: 5 in, 5 out]
        n244 = Unbundle By Name(w434) -> ("Column"=w431:i32, "Row"=w448:i32)
        n245 = property class="MCListbox (严格)"(reference=w443, "ActiveCell"=w434) -> (reference out=w442:refnum<vi>)  [unwired: 1 in, 1 out]
        n246 = local read "Size"() -> (w433:i32)
        n247 = Greater Or Equal To 0?(x=w448) -> (x >= 0?=w439:bool)
        n248 = Equal?(x=w431, y=5) -> (x = y?=w440:bool)
        n249 = Less?(x=w448, y=w433) -> (x < y?=w432:bool)
        n250 = property class="MCListbox (严格)"(reference=w442) -> (reference out=w435:refnum<vi>, "CellBG"=w437:u32)  [unwired: 1 in, 1 out]
        n251 = Compound Arithmetic op=AND(w440, w439, w432) -> (w441:bool)
        n252 = Index Array(array=w430, index=w448) -> (element=w444:i32)
        n253 = Index Array(array=w429, index=w448) -> (element=w446:i32)
        n254 = Index Array(array=w447, index=w448) -> (element=w449:i32)
        n255 = Not Equal?(x=w437, y=u32 6618880) -> (x != y?=w438:bool)
        n256 = Index Array(array=w428, index=w444) -> (element=w445:i16)
        n257 = And(x=w438, y=w441) -> (x .and. y?=w436:bool)
        n258 = case shown="真" w436 {
          selector: w436 -> [w458 w473]
          tunnel: w435 -> [w461 w477]
          tunnel: w431 -> [w457 _]
          tunnel: w445 -> [w452 w475]
          tunnel: w446 -> [w451 w474]
          tunnel: w448 -> [w453 _]
          tunnel: w449 -> [w450 w470]
          frame False {
            n259 = Not Equal?(x=w457, y=5) -> (x != y?=w454:bool)
            n260 = Equal?(x=w453, y=-1) -> (x = y?=w459:bool)
            n261 = Or(x=w454, y=w459) -> (x .or. y?=w455:bool)
            n262 = case shown="假" w455 {
              tunnel: w461 -> [w468 _]
              tunnel: w458 -> [w463 _]
              tunnel: w452 -> [w464 _]
              tunnel: w451 -> [w465 _]
              tunnel: w450 -> [w462 _]
              frame False {
                n263 = Boolean To (0,1)(Boolean=w463) -> (0, 1=w467:i16)
                n264 = call "DO Write Line.vi"("Value"=w467, "Line"=w465, "Port"=w462, "CardNumber"=w464) -> ("error out"=w466:errorcluster)  [unwired: 6 in, 1 out]
                n265 = property class="MCListbox (严格)"(reference=w468, "CellBG"=u32 3355443) -> ()  [unwired: 1 in, 2 out]
                n266 = call <vilib>:"Clear Errors.vi"("error in (no error)"=w466) -> ()  [unwired: 5 in, 2 out]
              }
              frame True {
              }
            }
          }
          frame True {
            n267 = Boolean To (0,1)(Boolean=w473) -> (0, 1=w472:i16)
            n268 = property class="MCListbox (严格)"(reference=w477, "CellBG"=u32 6618880) -> ()  [unwired: 1 in, 2 out]
            n269 = call "DO Write Line.vi"("Value"=w472, "Line"=w474, "Port"=w470, "CardNumber"=w475) -> ("error out"=w471:errorcluster)  [unwired: 6 in, 1 out]
            n270 = call <vilib>:"Clear Errors.vi"("error in (no error)"=w471) -> ()  [unwired: 5 in, 2 out]
          }
        }
      }
      event "HD Config Save": Value Change {
        n271 = event-data() -> ("NewVal"=w478:bool)  [unwired: 1 in]
        n272 = case shown="真" w478 {
          tunnel: w479 -> [_ w483]
          frame False {
          }
          frame True {
            n273 = call "Enter password"() -> ("Password"=w482:string)  [unwired: 17 in, 2 out]
            n274 = Equal?(x=w482, y="myzy@123") -> (x = y?=w480:bool)
            n275 = case shown="假" w480 {
              tunnel: w483 -> [_ w487]
              frame False {
                n276 = One Button Dialog(message="Password error" ("消息"), button name ("OK")="OK" ("按钮名称（“确定”）")) -> ()  [unwired: 1 out]
              }
              frame True {
                n277 = call "AMC Send Local Message.vi"("Message Name"="HD Config Save", "Message Queue in"=w487) -> ()  [unwired: 8 in, 2 out]
              }
            }
          }
        }
      }
      event "SW Config Save": Value Change {
        n278 = event-data() -> ("NewVal"=w489:bool)  [unwired: 1 in]
        n279 = case shown="真" w489 {
          tunnel: w488 -> [_ w493]
          frame False {
          }
          frame True {
            n280 = call "Enter password"() -> ("Password"=w492:string)  [unwired: 17 in, 2 out]
            n281 = Equal?(x=w492, y="myzy@123") -> (x = y?=w490:bool)
            n282 = case shown="真" w490 {
              tunnel: w493 -> [_ w496]
              frame False {
                n283 = One Button Dialog(message="Password error" ("消息"), button name ("OK")="OK" ("按钮名称（“确定”）")) -> ()  [unwired: 1 out]
              }
              frame True {
                n284 = call "AMC Send Local Message.vi"("Message Name"="SW Config Save", "Message Queue in"=w496) -> ()  [unwired: 8 in, 2 out]
              }
            }
          }
        }
      }
      event "Position Config Save": Value Change {
        n285 = event-data() -> ("NewVal"=w498:bool)  [unwired: 1 in]
        n286 = case shown="真" w498 {
          tunnel: w499 -> [_ w503]
          frame False {
          }
          frame True {
            n287 = call "Enter password"() -> ("Password"=w502:string)  [unwired: 17 in, 2 out]
            n288 = Equal?(x=w502, y="myzy@123") -> (x = y?=w500:bool)
            n289 = case shown="假" w500 {
              tunnel: w503 -> [_ w506]
              frame False {
                n290 = One Button Dialog(message="Password error" ("消息"), button name ("OK")="OK" ("按钮名称（“确定”）")) -> ()  [unwired: 1 out]
              }
              frame True {
                n291 = call "AMC Send Local Message.vi"("Message Name"="Position Config Save", "Message Queue in"=w506) -> ()  [unwired: 8 in, 2 out]
              }
            }
          }
        }
      }
      event "FCO Model5_Read": Value Change {
        n292 = event-data() -> ("NewVal"=w508:bool)  [unwired: 1 in]
        n293 = case shown="真" w508 {
          tunnel: w509 -> [_ w510]
          frame False {
          }
          frame True {
            n294 = call "AMC Send Local Message.vi"("Message Name"="FCO_Read", "Message Queue in"=w510) -> ()  [unwired: 8 in, 2 out]
          }
        }
      }
      event "Zero pressure": Value Change {
        n295 = event-data() -> ("NewVal"=w512:bool)  [unwired: 1 in]
        n296 = case shown="真" w512 {
          tunnel: w513 -> [_ w517]
          frame False {
          }
          frame True {
            n297 = call "Enter password"() -> ("Password"=w516:string)  [unwired: 17 in, 2 out]
            n298 = Equal?(x=w516, y="myzy@123") -> (x = y?=w514:bool)
            n299 = case shown="假" w514 {
              tunnel: w517 -> [_ w520]
              frame False {
                n300 = One Button Dialog(message="Password error" ("消息"), button name ("OK")="OK" ("按钮名称（“确定”）")) -> ()  [unwired: 1 out]
              }
              frame True {
                n301 = call "AMC Send Local Message.vi"("Message Name"="FCO_Zero_pressure", "Message Queue in"=w520) -> ()  [unwired: 8 in, 2 out]
              }
            }
          }
        }
      }
      event "PW3336": Value Change {
        n302 = event-data() -> ("NewVal"=w522:bool)  [unwired: 1 in]
        n303 = case shown="真" w522 {
          tunnel: w523 -> [_ w524]
          frame False {
          }
          frame True {
            n304 = call "AMC Send Local Message.vi"("Message Name"="PW3336_Read", "Message Queue in"=w524) -> ()  [unwired: 8 in, 2 out]
          }
        }
      }
      event "Lefoo": Value Change {
        n305 = event-data() -> ("NewVal"=w526:bool)  [unwired: 1 in]
        n306 = case shown="真" w526 {
          tunnel: w527 -> [_ w528]
          frame False {
          }
          frame True {
            n307 = call "AMC Send Local Message.vi"("Message Name"="Lefoo_Read", "Message Queue in"=w528) -> ()  [unwired: 8 in, 2 out]
          }
        }
      }
      event "Read_NFC": Value Change {
        n308 = event-data() -> ("NewVal"=w532:bool)  [unwired: 1 in]
        n309 = case shown="真" w532 {
          tunnel: w533 -> [_ w534]
          frame False {
          }
          frame True {
            n310 = call "AMC Send Local Message.vi"("Message Name"="Read_NFC_Read", "Message Queue in"=w534) -> ()  [unwired: 8 in, 2 out]
          }
        }
        n311 = property on="DataTag" class="Str"("Value"="") -> ()  [unwired: 2 in, 2 out]
        n312 = property on="UID" class="Str"("Value"="" ("UID")) -> ()  [unwired: 2 in, 2 out]
      }
      event "DC": Value Change {
        n313 = event-data() -> ("NewVal"=w536:bool)  [unwired: 1 in]
        n314 = case shown="真" w536 {
          tunnel: w537 -> [_ w538]
          frame False {
          }
          frame True {
            n315 = call "AMC Send Local Message.vi"("Message Name"="DC_Read", "Message Queue in"=w538) -> ()  [unwired: 8 in, 2 out]
          }
        }
      }
      event "DC_Set": Value Change {
        n316 = event-data() -> ("NewVal"=w540:bool)  [unwired: 1 in]
        n317 = case shown="真" w540 {
          tunnel: w541 -> [_ w542]
          frame False {
          }
          frame True {
            n318 = call "AMC Send Local Message.vi"("Message Name"="DC_Set", "Message Queue in"=w542) -> ()  [unwired: 8 in, 2 out]
          }
        }
      }
      event "DC_Power_ON/OFF": Value Change {
        n319 = event-data() -> ("NewVal"=w544:bool)  [unwired: 1 in]
        n320 = case shown="真" w544 {
          tunnel: w545 -> [w546 w549]
          frame False {
            n321 = call "AMC Send Local Message.vi"("Message Name"="DC_Power_OFF", "Message Queue in"=w546) -> ()  [unwired: 8 in, 2 out]
          }
          frame True {
            n322 = property on="Relay_ON/OFF" class="Bool (严格)"() -> ("Value"=w548:bool)  [unwired: 2 in, 2 out]
            n323 = case shown="假" w548 {
              tunnel: w549 -> [_ w553]
              frame False {
                n324 = property on="DC_Power_ON/OFF" class="Bool (严格)"("Value"=FALSE ("DC_Power_ON/OFF")) -> ()  [unwired: 2 in, 2 out]
                n325 = One Button Dialog(message="Please Relay_ON first" ("消息"), button name ("OK")="OK" ("按钮名称（“确定”）")) -> ()  [unwired: 1 out]
              }
              frame True {
                n326 = call "AMC Send Local Message.vi"("Message Name"="DC_Power_ON", "Message Queue in"=w553) -> ()  [unwired: 8 in, 2 out]
              }
            }
          }
        }
      }
      event "Relay_ON/OFF": Value Change {
        n327 = event-data() -> ("NewVal"=w555:bool)  [unwired: 1 in]
        n328 = case shown="假" w555 {
          tunnel: w556 -> [w558 w564]
          frame False {
            n329 = property on="DC_Power_ON/OFF" class="Bool (strict)"() -> ("Value"=w557:bool)  [unwired: 2 in, 2 out]
            n330 = case shown="真" w557 {
              tunnel: w558 -> [w559 _]
              frame False {
                n331 = call "AMC Send Local Message.vi"("Message Name"="Relay_OFF", "Message Queue in"=w559) -> ()  [unwired: 8 in, 2 out]
              }
              frame True {
                n332 = property on="Relay_ON/OFF" class="Bool (严格)"("Value"=TRUE ("Relay_ON/OFF")) -> ()  [unwired: 2 in, 2 out]
                n333 = One Button Dialog(message="Please DC_Power_OFF first" ("消息"), button name ("OK")="OK" ("按钮名称（“确定”）")) -> ()  [unwired: 1 out]
              }
            }
          }
          frame True {
            n334 = call "AMC Send Local Message.vi"("Message Name"="Relay_ON", "Message Queue in"=w564) -> ()  [unwired: 8 in, 2 out]
          }
        }
      }
      event "Home": Value Change {
        n335 = event-data() -> ("NewVal"=w567:bool)  [unwired: 1 in]
        n336 = case shown="真" w567 {
          tunnel: w566 -> [_ w571]
          frame False {
          }
          frame True {
            n337 = call "Enter password"() -> ("Password"=w570:string)  [unwired: 17 in, 2 out]
            n338 = Equal?(x=w570, y="myzy@123") -> (x = y?=w568:bool)
            n339 = case shown="假" w568 {
              tunnel: w571 -> [_ w574]
              frame False {
                n340 = One Button Dialog(message="Password error" ("消息"), button name ("OK")="OK" ("按钮名称（“确定”）")) -> ()  [unwired: 1 out]
              }
              frame True {
                n341 = call "AMC Send Local Message.vi"("Message Name"="Home", "Message Queue in"=w574) -> ()  [unwired: 8 in, 2 out]
              }
            }
          }
        }
      }
      event "Reset": Value Change {
        n342 = event-data() -> ("NewVal"=w577:bool)  [unwired: 1 in]
        n343 = case shown="真" w577 {
          tunnel: w576 -> [_ w581]
          frame False {
          }
          frame True {
            n344 = call "Enter password"() -> ("Password"=w580:string)  [unwired: 17 in, 2 out]
            n345 = Equal?(x=w580, y="myzy@123") -> (x = y?=w578:bool)
            n346 = case shown="假" w578 {
              tunnel: w581 -> [_ w584]
              frame False {
                n347 = One Button Dialog(message="Password error" ("消息"), button name ("OK")="OK" ("按钮名称（“确定”）")) -> ()  [unwired: 1 out]
              }
              frame True {
                n348 = call "AMC Send Local Message.vi"("Message Name"="Reset", "Message Queue in"=w584) -> ()  [unwired: 8 in, 2 out]
              }
            }
          }
        }
      }
      event "Set_Speed": Value Change {
        n349 = event-data() -> ("NewVal"=w587:bool)  [unwired: 1 in]
        n350 = case shown="真" w587 {
          tunnel: w586 -> [_ w591]
          frame False {
          }
          frame True {
            n351 = call "Enter password"() -> ("Password"=w590:string)  [unwired: 17 in, 2 out]
            n352 = Equal?(x=w590, y="myzy@123") -> (x = y?=w588:bool)
            n353 = case shown="假" w588 {
              tunnel: w591 -> [_ w594]
              frame False {
                n354 = One Button Dialog(message="Password error" ("消息"), button name ("OK")="OK" ("按钮名称（“确定”）")) -> ()  [unwired: 1 out]
              }
              frame True {
                n355 = call "AMC Send Local Message.vi"("Message Name"="Set_Speed", "Message Queue in"=w594) -> ()  [unwired: 8 in, 2 out]
              }
            }
          }
        }
      }
      event "Stop": Value Change {
        n356 = event-data() -> ("NewVal"=w597:bool)  [unwired: 1 in]
        n357 = case shown="真" w597 {
          tunnel: w596 -> [_ w601]
          frame False {
          }
          frame True {
            n358 = call "Enter password"() -> ("Password"=w600:string)  [unwired: 17 in, 2 out]
            n359 = Equal?(x=w600, y="myzy@123") -> (x = y?=w598:bool)
            n360 = case shown="假" w598 {
              tunnel: w601 -> [_ w604]
              frame False {
                n361 = One Button Dialog(message="Password error" ("消息"), button name ("OK")="OK" ("按钮名称（“确定”）")) -> ()  [unwired: 1 out]
              }
              frame True {
                n362 = call "AMC Send Local Message.vi"("Message Name"="Stop", "Message Queue in"=w604) -> ()  [unwired: 8 in, 2 out]
              }
            }
          }
        }
      }
      event "GoPosition": Value Change {
        n363 = event-data() -> ("NewVal"=w607:bool)  [unwired: 1 in]
        n364 = case shown="真" w607 {
          tunnel: w606 -> [_ w611]
          frame False {
          }
          frame True {
            n365 = call "Enter password"() -> ("Password"=w610:string)  [unwired: 17 in, 2 out]
            n366 = Equal?(x=w610, y="myzy@123") -> (x = y?=w608:bool)
            n367 = case shown="假" w608 {
              tunnel: w611 -> [_ w614]
              frame False {
                n368 = One Button Dialog(message="Password error" ("消息"), button name ("OK")="OK" ("按钮名称（“确定”）")) -> ()  [unwired: 1 out]
              }
              frame True {
                n369 = call "AMC Send Local Message.vi"("Message Name"="GoPosition", "Message Queue in"=w614) -> ()  [unwired: 8 in, 2 out]
              }
            }
          }
        }
      }
      event "Servo_On": Value Change {
        n370 = event-data() -> ("NewVal"=w617:bool)  [unwired: 1 in]
        n371 = case shown="真" w617 {
          tunnel: w616 -> [_ w621]
          frame False {
          }
          frame True {
            n372 = call "Enter password"() -> ("Password"=w620:string)  [unwired: 17 in, 2 out]
            n373 = Equal?(x=w620, y="myzy@123") -> (x = y?=w618:bool)
            n374 = case shown="假" w618 {
              tunnel: w621 -> [_ w624]
              frame False {
                n375 = One Button Dialog(message="Password error" ("消息"), button name ("OK")="OK" ("按钮名称（“确定”）")) -> ()  [unwired: 1 out]
              }
              frame True {
                n376 = call "AMC Send Local Message.vi"("Message Name"="Servo_On", "Message Queue in"=w624) -> ()  [unwired: 8 in, 2 out]
              }
            }
          }
        }
      }
      event "Servo_Off": Value Change {
        n377 = event-data() -> ("NewVal"=w627:bool)  [unwired: 1 in]
        n378 = case shown="真" w627 {
          tunnel: w626 -> [_ w631]
          frame False {
          }
          frame True {
            n379 = call "Enter password"() -> ("Password"=w630:string)  [unwired: 17 in, 2 out]
            n380 = Equal?(x=w630, y="myzy@123") -> (x = y?=w628:bool)
            n381 = case shown="假" w628 {
              tunnel: w631 -> [_ w634]
              frame False {
                n382 = One Button Dialog(message="Password error" ("消息"), button name ("OK")="OK" ("按钮名称（“确定”）")) -> ()  [unwired: 1 out]
              }
              frame True {
                n383 = call "AMC Send Local Message.vi"("Message Name"="Servo_Off", "Message Queue in"=w634) -> ()  [unwired: 8 in, 2 out]
              }
            }
          }
        }
      }
      event "Set EOL": Value Change {
        n384 = event-data() -> ("NewVal"=w637:bool)  [unwired: 1 in]
        n385 = case shown="真" w637 {
          tunnel: w636 -> [_ w641]
          frame False {
          }
          frame True {
            n386 = call "Enter password"() -> ("Password"=w640:string)  [unwired: 17 in, 2 out]
            n387 = Equal?(x=w640, y="myzy@123") -> (x = y?=w638:bool)
            n388 = case shown="假" w638 {
              tunnel: w641 -> [_ w644]
              frame False {
                n389 = One Button Dialog(message="Password error" ("消息"), button name ("OK")="OK" ("按钮名称（“确定”）")) -> ()  [unwired: 1 out]
              }
              frame True {
                n390 = call "AMC Send Local Message.vi"("Message Name"="Set_EOL", "Message Queue in"=w644) -> ()  [unwired: 8 in, 2 out]
              }
            }
          }
        }
      }
      event "Production Mode": Value Change {
        n391 = event-data() -> ("NewVal"=w648:bool)  [unwired: 1 in]
        n392 = case shown="真" w648 {
          tunnel: w647 -> [_ w650]
          tunnel: [_ TRUE ("停止")] -> w646
          frame False {
          }
          frame True {
            n393 = call "AMC Send Local Message.vi"("Message Name"="PrductionMode", "Message Queue in"=w650) -> ()  [unwired: 8 in, 2 out]
          }
        }
      }
    }
    n394 = call "Exit.vi"("Step"=enum16{"Initial", "Write", "Read"}."Read") -> ("Exit Out"=w390:bool)  [unwired: 9 in, 1 out]
    n395 = Or(x=w387, y=w390) -> (x .or. y?=w391:bool)
  }
